vi "Read comments from sxp-file.vi"(7 "Comment character":string="!", 8 "error in (no error)":errorcluster, 11 "file path":path) -> (0 "error out":errorcluster, 2 "Comment lines":string[](array[string]), 3 "file path out":path)   [LabVIEW 2020]
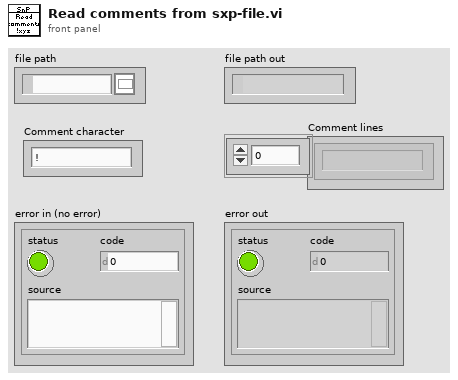
[diagram p1: front panel]
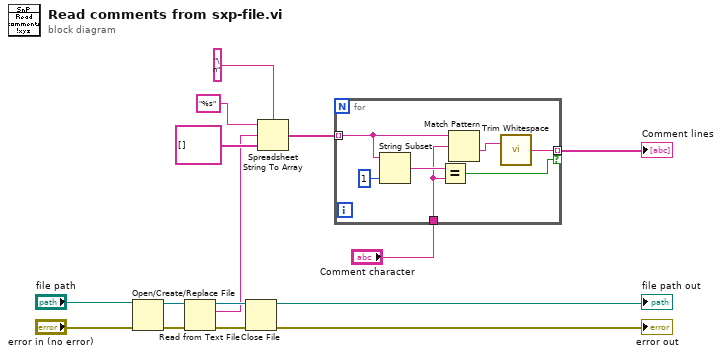
[diagram p0: block diagram]
diagram:
  n1 = Open/Create/Replace File(file path (use dialog)="file path", error in="error in (no error)") -> (refnum out=w8:refnum<file>, error out=w7:errorcluster)  [unwired: 4 in, 1 out]
  n2 = Read from Text File(file (use dialog)=w8, error in=w7) -> (refnum out=w6:refnum<file>, text=w4:string, error out=w5:errorcluster)  [unwired: 2 in, 1 out]
  n3 = Close File(refnum=w6, error in=w5) -> (path=→"file path out":path, error out=→"error out":errorcluster)
  n4 = Spreadsheet String To Array(delimiter (Tab)="\n", format string="%s", spreadsheet string=w4, array type (2D Dbl)=string[] []) -> (array=w3:string[])
  n5 = for {
    tunnel: w3 -> [w18] mode=indexing
    tunnel: [w16] -> w12 mode=indexing if=w20
    tunnel: "Comment character" -> [w19]
    n6 = String Subset(string=w18, length (rest)=1 ("length (rest)")) -> (substring=w21:string)  [unwired: 1 in]
    n7 = Equal?(x=w21, y=w19) -> (x = y?=w20:bool)
    n8 = Match Pattern(string=w18, regular expression=w19) -> (after substring=w17:string)  [unwired: 1 in, 3 out]
    n9 = call <vilib>:"Trim Whitespace.vi"("string"=w17) -> ("trimmed string"=w16:string)  [unwired: 1 in]
  }
  "Comment lines" <- w12
